vi "UI_enable.vi"(8 "error in":errorcluster, 10 "Boolean":bool, 11 "?":T1) -> (0 "error out":errorcluster)   [LabVIEW 2020]
uses:
  controls/VI_ref.ctl
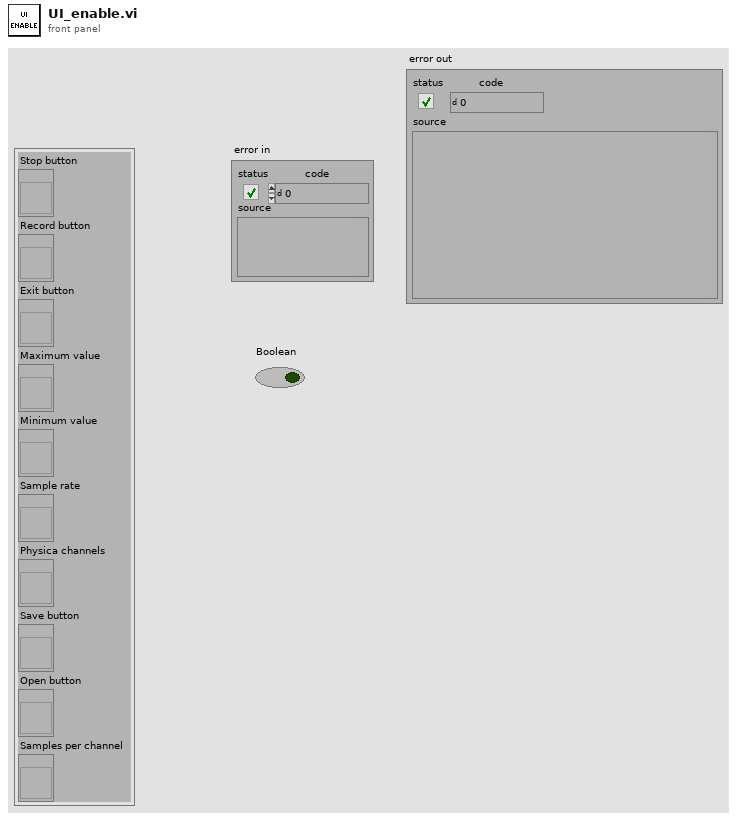
[diagram p1: front panel]
types:
  T1 = typedef "VI_ref.ctl" = cluster{"Stop button":refnum<vi>, "Record button":refnum<vi>, "Exit button":refnum<vi>, "Maximum value":refnum<vi>, "Minimum value":refnum<vi>, "Sample rate":refnum<vi>, "Physica channels":refnum<vi>, "Save button":refnum<vi>, "Open button":refnum<vi>, "Samples per channel":refnum<vi>}
  T2 = enum8{"Enabled", "Disabled", "Disabled and Grayed Out"}
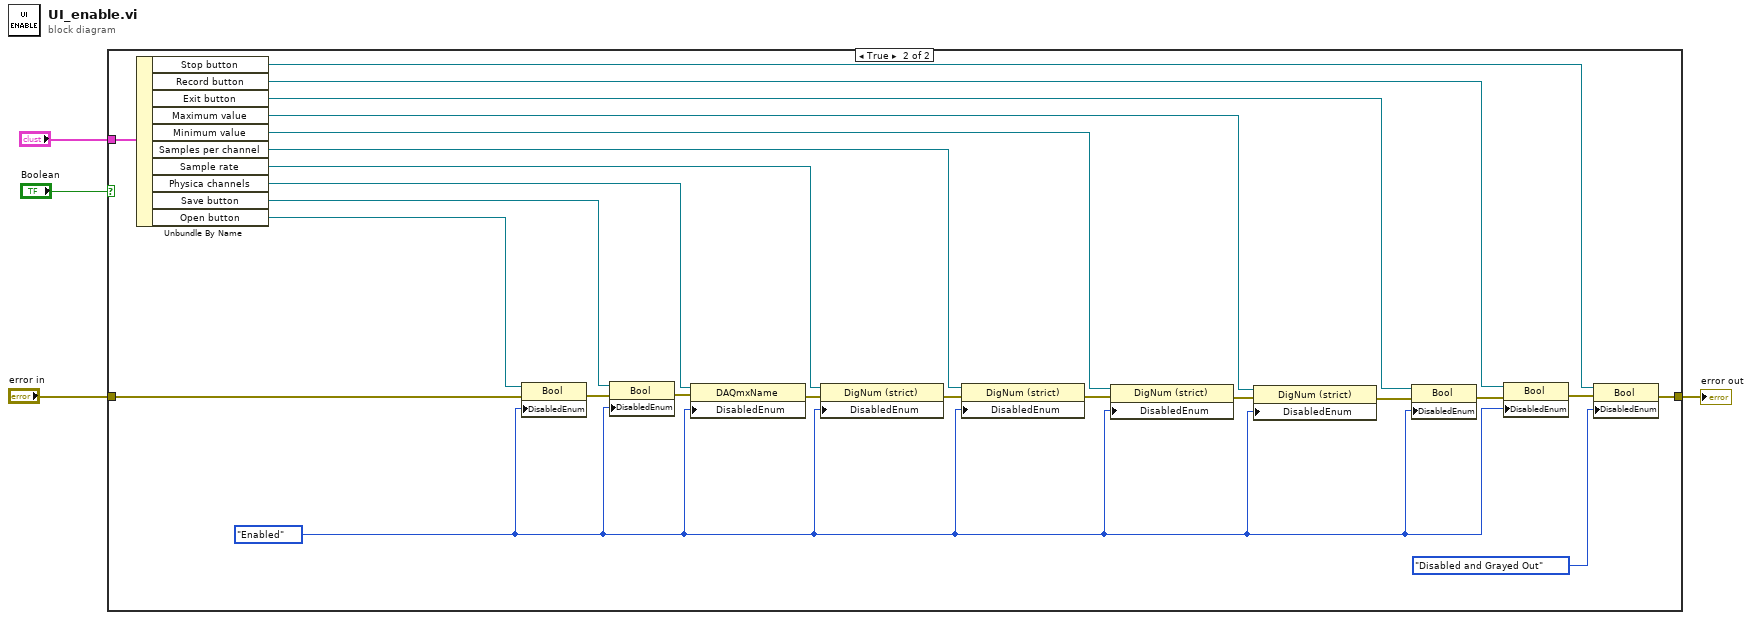
[diagram p0: block diagram]
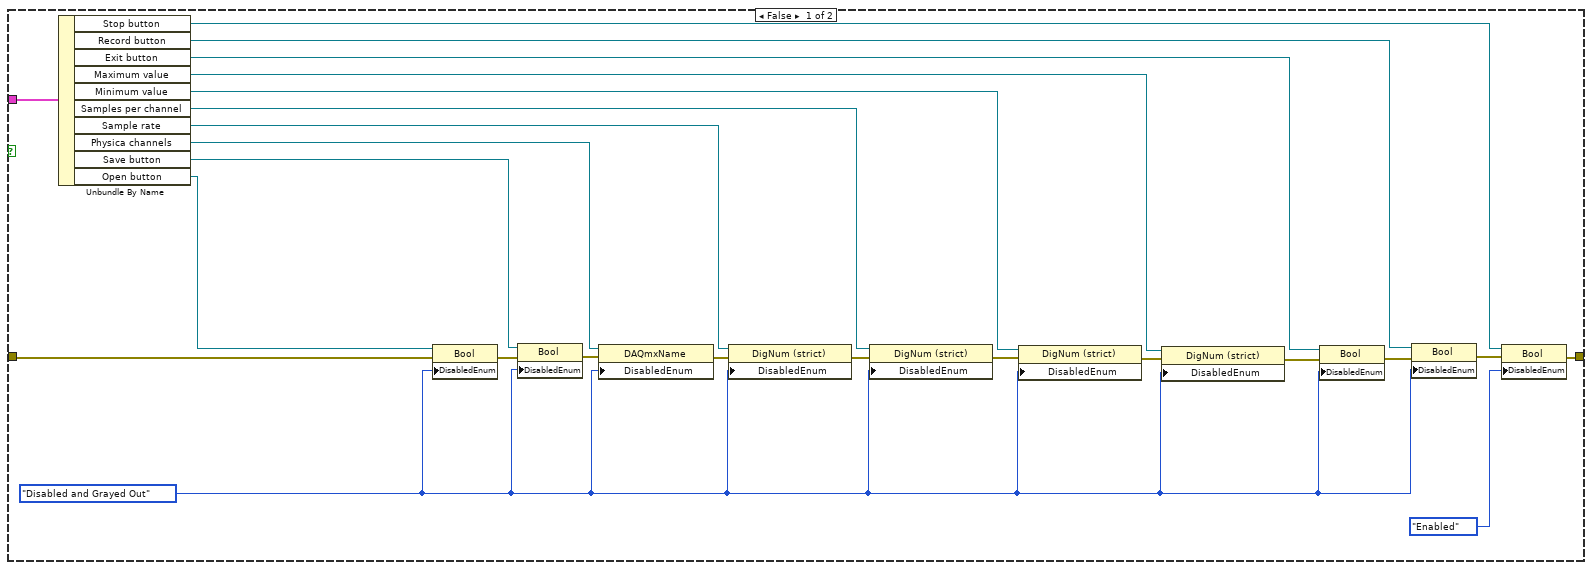
[diagram p2: hidden frame]
diagram:
  n1 = case shown="True" "Boolean" {
    tunnel: "error in" -> [w5 w32]
    tunnel: "?" -> [w12 w35]
    tunnel: [w11 w36] -> w1
    frame False {
      w6 = T2."Disabled and Grayed Out" ("Disabled")
      n2 = Unbundle By Name(w12) -> ("Stop button"=w21:refnum<vi>, "Record button"=w20:refnum<vi>, "Exit button"=w19:refnum<vi>, "Maximum value"=w18:refnum<vi>, "Minimum value"=w17:refnum<vi>, "Samples per channel"=w16:refnum<vi>, "Sample rate"=w15:refnum<vi>, "Physica channels"=w14:refnum<vi>, "Save button"=w10:refnum<vi>, "Open button"=w9:refnum<vi>)
      n3 = property on="Property Node" class="Bool"(reference=w9, error in=w5, "DisabledEnum"=w6) -> (error out=w8:errorcluster)  [unwired: 1 out]
      n4 = property on="Property Node" class="Bool"(reference=w10, error in=w8, "DisabledEnum"=w6) -> (error out=w7:errorcluster)  [unwired: 1 out]
      n5 = property on="Property Node" class="DAQmxName"(reference=w14, error in=w7, "DisabledEnum"=w6) -> (error out=w22:errorcluster)  [unwired: 1 out]
      n6 = property on="Property Node" class="DigNum (strict)"(reference=w15, error in=w22, "DisabledEnum"=w6) -> (error out=w23:errorcluster)  [unwired: 1 out]
      n7 = property on="Property Node" class="DigNum (strict)"(reference=w16, error in=w23, "DisabledEnum"=w6) -> (error out=w24:errorcluster)  [unwired: 1 out]
      n8 = property on="Property Node" class="DigNum (strict)"(reference=w17, error in=w24, "DisabledEnum"=w6) -> (error out=w25:errorcluster)  [unwired: 1 out]
      n9 = property on="Property Node" class="DigNum (strict)"(reference=w18, error in=w25, "DisabledEnum"=w6) -> (error out=w26:errorcluster)  [unwired: 1 out]
      n10 = property on="Property Node" class="Bool"(reference=w19, error in=w26, "DisabledEnum"=w6) -> (error out=w27:errorcluster)  [unwired: 1 out]
      n11 = property on="Property Node" class="Bool"(reference=w20, error in=w27, "DisabledEnum"=w6) -> (error out=w28:errorcluster)  [unwired: 1 out]
      n12 = property on="Property Node" class="Bool"(reference=w21, error in=w28, "DisabledEnum"=T2."Enabled" ("Disabled")) -> (error out=w11:errorcluster)  [unwired: 1 out]
    }
    frame True {
      w30 = T2."Enabled" ("Disabled")
      n13 = Unbundle By Name(w35) -> ("Stop button"=w45:refnum<vi>, "Record button"=w46:refnum<vi>, "Exit button"=w47:refnum<vi>, "Maximum value"=w48:refnum<vi>, "Minimum value"=w49:refnum<vi>, "Samples per channel"=w50:refnum<vi>, "Sample rate"=w51:refnum<vi>, "Physica channels"=w52:refnum<vi>, "Save button"=w34:refnum<vi>, "Open button"=w33:refnum<vi>)
      n14 = property on="Property Node" class="Bool"(reference=w33, error in=w32, "DisabledEnum"=w30) -> (error out=w31:errorcluster)  [unwired: 1 out]
      n15 = property on="Property Node" class="Bool"(reference=w34, error in=w31, "DisabledEnum"=w30) -> (error out=w29:errorcluster)  [unwired: 1 out]
      n16 = property on="Property Node" class="DAQmxName"(reference=w52, error in=w29, "DisabledEnum"=w30) -> (error out=w43:errorcluster)  [unwired: 1 out]
      n17 = property on="Property Node" class="DigNum (strict)"(reference=w51, error in=w43, "DisabledEnum"=w30) -> (error out=w42:errorcluster)  [unwired: 1 out]
      n18 = property on="Property Node" class="DigNum (strict)"(reference=w50, error in=w42, "DisabledEnum"=w30) -> (error out=w41:errorcluster)  [unwired: 1 out]
      n19 = property on="Property Node" class="DigNum (strict)"(reference=w49, error in=w41, "DisabledEnum"=w30) -> (error out=w40:errorcluster)  [unwired: 1 out]
      n20 = property on="Property Node" class="DigNum (strict)"(reference=w48, error in=w40, "DisabledEnum"=w30) -> (error out=w39:errorcluster)  [unwired: 1 out]
      n21 = property on="Property Node" class="Bool"(reference=w47, error in=w39, "DisabledEnum"=w30) -> (error out=w38:errorcluster)  [unwired: 1 out]
      n22 = property on="Property Node" class="Bool"(reference=w46, error in=w38, "DisabledEnum"=w30) -> (error out=w37:errorcluster)  [unwired: 1 out]
      n23 = property on="Property Node" class="Bool"(reference=w45, error in=w37, "DisabledEnum"=T2."Disabled and Grayed Out" ("Disabled")) -> (error out=w36:errorcluster)  [unwired: 1 out]
    }
  }
  "error out" <- w1
